vi "Configure Right Click Menu.vi"(7 "Table Reference":refnum<vi>, 8 "error in (no error)":errorcluster, 10 "Coords":T1, 11 "Menu in":refnum<k9>) -> (0 "error out":errorcluster)   [LabVIEW 2016, in "Assert API Components.lvlib" / "Assert Display.lvlib" / "Service Config Display.lvlib" / "Service Config Display.lvclass"]
doc: "Configures the services table right click menu when the event is triggered"
uses:
  Service Config Display.lvclass
  <vilib>/Utility/miscctls.llb/LVPoint32TypeDef.ctl
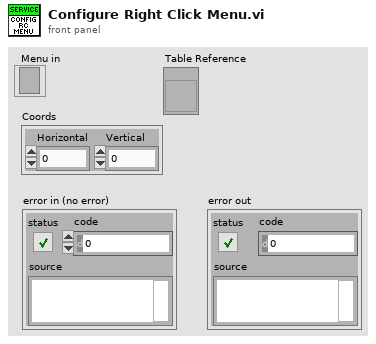
[diagram p1: front panel]
types:
  T1 = typedef "LVPoint32TypeDef.ctl" = cluster{"Horizontal":i32, "Vertical":i32}
  T2 = typedef "LVRowAndColumnTypeDef.ctl" = cluster{"Row":i32, "Column":i32}
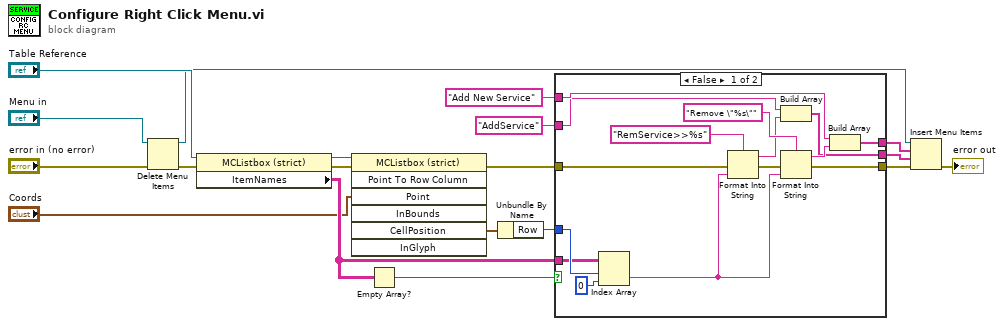
[diagram p0: block diagram]
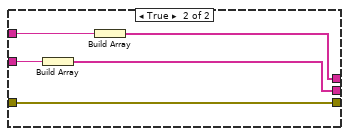
[diagram p2: hidden frame]
diagram:
  n1 = Delete Menu Items(6:"error in (no error)", 9:"Menu in") -> (0:w10:errorcluster, 3:w9:refnum<k9>)  [unwired: 2 in]
  n2 = property class="MCListbox (strict)"(reference="Table Reference", error in=w10) -> (reference out=w5:refnum<vi>, error out=w4:errorcluster, "ItemNames"=w6:string[][])
  n3 = invoke class="MCListbox (strict)" method="Point To Row Column"(reference=w5, error in=w4, "Point"="Coords") -> (error out=w3:errorcluster, "CellPosition"=w1:T2)  [unwired: 4 in, 5 out]
  n4 = Empty Array?(array=w6) -> (empty?=w8:bool)
  n5 = Unbundle By Name(w1) -> ("Row"=w7:i32)
  n6 = case shown="False" w8 {
    tunnel: "Add New Service" -> [w34 w37]
    tunnel: "AddService" -> [w32 w38]
    tunnel: [w31 w35] -> w13
    tunnel: [w30 w36] -> w12
    tunnel: w3 -> [w26 w39]
    tunnel: [w29 w39] -> w11
    tunnel: w7 -> [w23 _]
    tunnel: w6 -> [w22 _]
    frame False {
      n7 = Index Array(array=w22, index (row)=w23, index (col)=0 ("disabled index (col)")) -> (element=w20:string)
      n8 = Format Into String(format string="RemService>>%s", error in=w26, w20) -> (resulting string=w21:string, error out=w27:errorcluster)  [unwired: 1 in]
      n9 = Build Array(w32, w21) -> (w31:string[])
      n10 = Format Into String(format string="Remove \"%s\"", error in=w27, w20) -> (resulting string=w33:string, error out=w29:errorcluster)  [unwired: 1 in]
      n11 = Build Array(w34, w33) -> (w30:string[])
    }
    frame True {
      n12 = Build Array(w38) -> (w35:string[])
      n13 = Build Array(w37) -> (w36:string[])
    }
  }
  n14 = Insert Menu Items(6:w11, 7:w13, 8:w12, 9:w9) -> (0:→"error out":errorcluster)  [unwired: 2 in, 2 out]
